vi "Rotate Angle in Radians.vi"   [LabVIEW 2017, in "NI_Robotics Utilities.lvlib"]
doc: "This VI is deprecated. Use <vi.lib>\\Analysis\\coordinate.llb\\Angle Rotation.vi instead."
uses:
  <vilib>/robotics/Utilities/NI_Robotics Utilities.lvlib
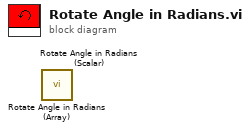
[diagram p0: block diagram]
diagram:
  n1 = call <vilib>:"Rotate Angle in Radians (Array).vi"() -> ()  [unwired: 11 in, 1 out]
  n2 = call <vilib>:"Rotate Angle in Radians (Scalar).vi"() -> ()  [unwired: 11 in, 1 out]
